vi "Fill DataTable (column array).vi"(8 "error in (no error)":errorcluster, 10 "columns":T1[](array[typedef]), 11 "JMP DataTable":refnum<k7>) -> (0 "error out":errorcluster, 3 "JMP data table out":refnum<k7>)   [LabVIEW 2019, in "JMP Automation.lvlib"]
doc: "Add columns with their coresponding data to a DataDable"
uses:
  <instrlib>/LV_JMP_bridge/JMP Automation.lvlib
  <instrlib>/LV_JMP_bridge/JMP Column.ctl
  <instrlib>/LV_JMP_bridge/JMP Column Header.ctl
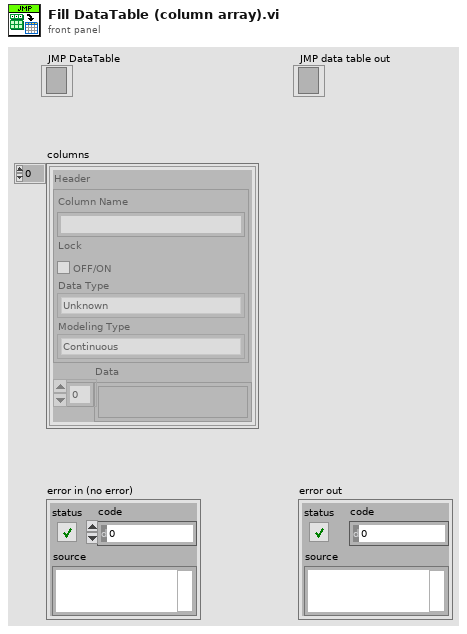
[diagram p1: front panel]
types:
  T1 = typedef "JMP Automation.lvlib/JMP Column.ctl" = cluster{"Header":T2, "Data":variant[]}
  T2 = typedef "JMP Automation.lvlib/JMP Column Header.ctl" = cluster{"Column Name":string, "Lock":bool, "Data Type":enum16{"Unknown", "Numeric", "Character", "RowState"}, "Modeling Type":enum16{"Continuous", "Ordinal", "Nominal"}}
  T3 = enum16{"Unknown", "Numeric", "Character", "RowState"}
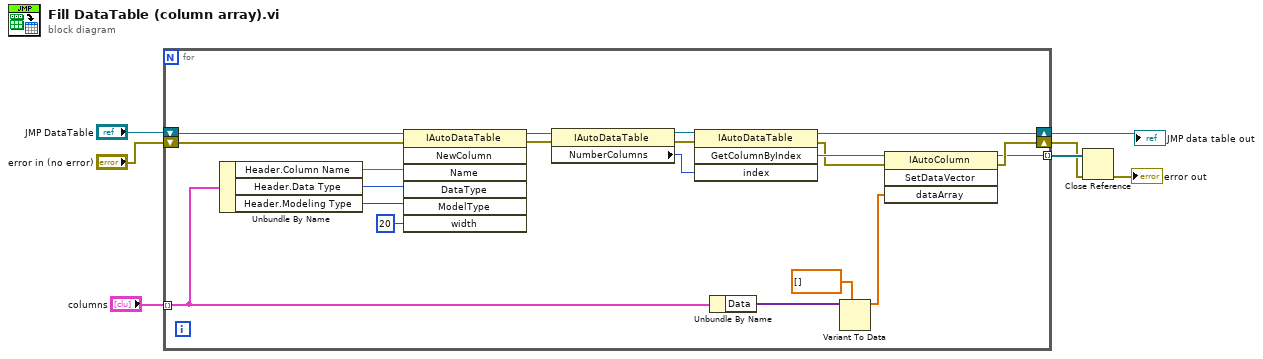
[diagram p0: block diagram]
diagram:
  n1 = for {
    shift-right: [w25] -> w7
    shift-left: "JMP DataTable" -> [w27]
    shift-right: [w18] -> w4
    shift-left: "error in (no error)" -> [w26]
    tunnel: "columns" -> [w17] mode=indexing
    tunnel: [w13] -> w5 mode=indexing
    n2 = Unbundle By Name(w17) -> ("Header.Column Name"=w19:string, "Header.Data Type"=w22:T3, "Header.Modeling Type"=w21:enum16{"Continuous", "Ordinal", "Nominal"})
    n3 = invoke class="IAutoDataTable" method="NewColumn"(reference=w27, error in=w26, "Name"=w19, "DataType"=w22, "ModelType"=w21, "width"=i16 20) -> (reference out=w9:refnum<k7>, error out=w8:errorcluster)  [unwired: 1 in, 5 out]
    n4 = property class="IAutoDataTable"(reference=w9, error in=w8) -> (reference out=w12:refnum<k7>, error out=w11:errorcluster, "NumberColumns"=w10:i32)
    n5 = invoke class="IAutoDataTable" method="GetColumnByIndex"(reference=w12, error in=w11, "index"=w10) -> (reference out=w25:refnum<k7>, error out=w23:errorcluster, "GetColumnByIndex"=w24:refnum<k7>)  [unwired: 1 in, 1 out]
    n6 = Unbundle By Name(w17) -> ("Data"=w15:variant[])
    n7 = Variant To Data(type=dbl[] [], Variant=w15) -> (data=w14:dbl[])  [unwired: 1 in, 1 out]
    n8 = invoke class="IAutoColumn" method="SetDataVector"(reference=w24, error in=w23, "dataArray"=w14) -> (reference out=w13:refnum<k7>, error out=w18:errorcluster)  [unwired: 1 in, 2 out]
  }
  "JMP data table out" <- w7
  n9 = Close Reference(reference=w5, error in (no error)=w4) -> (error out=→"error out":errorcluster)
